vi "Modbus Master Example.vi"() -> ()   [LabVIEW 2021]
doc: "An example of the modbus master functionality."
uses:
  API/Master/Modbus Master.lvclass
  Master Function Definition/Read Device ID code.ctl
  Data Model/Device Data Model.lvclass
  API/Wrapper/API Main.lvlib
panel:
  in  "Stop Button":bool
  in  "Port":u16=502
  in  "Set Holding Registers":bool
  in  "Set Coils":bool
  in  "Fetch Discrete Inputs":bool
  in  "Fetch Input Registers":bool
  in  "Fetch Basic Objects":bool
  out "Basic Objects":string[](array[string])
  out "Status":string
  in  "Disconnect":bool
  in  "Connect":bool
  in  "Holding Registers":u16[](array[numeric])=[0, 0, 0, 0, 0, 0, 0, 0]
  out "Input Registers":u16[](array[numeric])
  in  "Coils":bool[](array[boolean])=[FALSE, FALSE, FALSE, FALSE, FALSE, FALSE, FALSE, FALSE]
  out "Discrete Inputs":bool[](array[boolean])
  in  "Slave Address":string="localhost"
  # "Coils are the boolean outputs of a modbus device. This example allows you to set the first 8 outputs."
  # "Holding Registers are the integer outputs of a modbus device. This example allows you to set the first 8 outputs."
  # "Modbus devices can also store objects in their memory, which are variable length strings. This example requests the basic level of objects."
  # "Discrete inputs are the boolean inputs of a modbus device. This example allows you to read the first 8 inputs."
  # "Input Registers are the integer inputs of a modbus device. This example allows you to read the first 8 inputs."
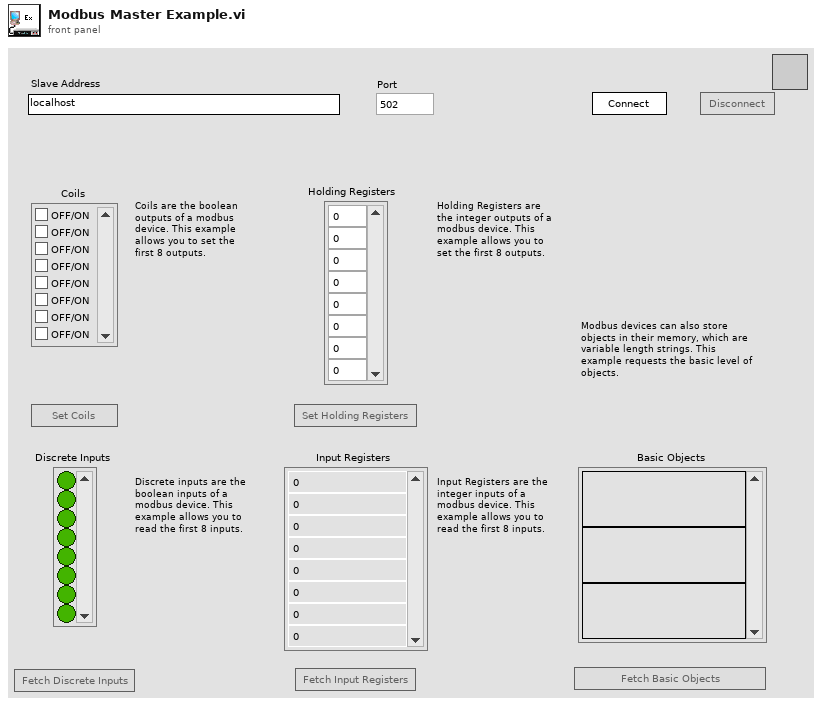
[diagram p1: front panel]
types:
  T1 = enum8{"Enabled", "Disabled", "Disabled and Grayed Out"}
  T2 = typedef "Device Data Model.lvclass/Read Device ID code.ctl" = enum8{"Read Basic", "Read Regular", "Read Extended", "Read Specific"}
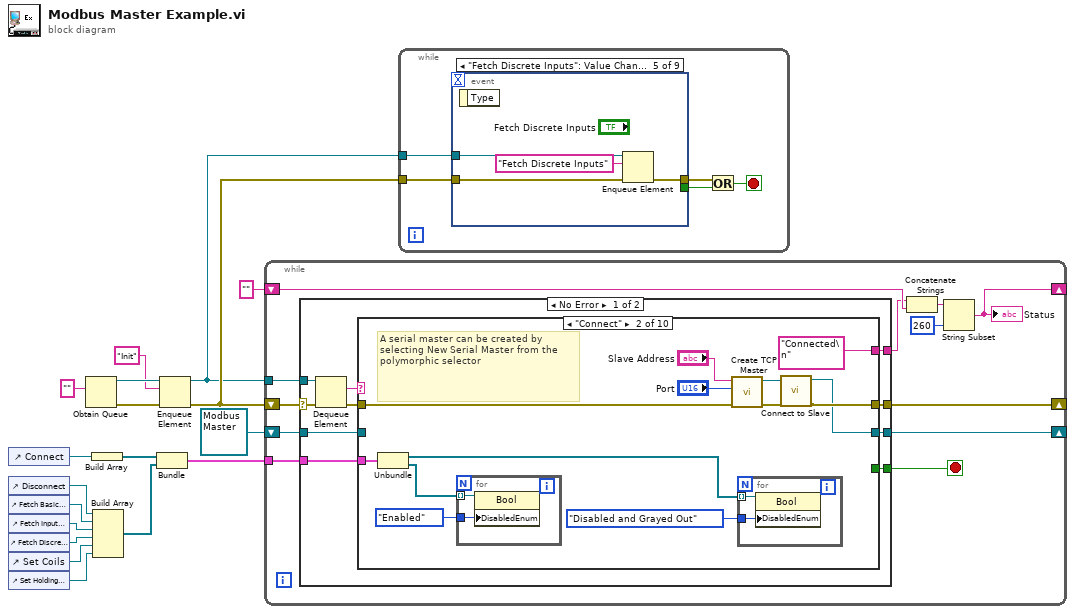
[diagram p0: block diagram]
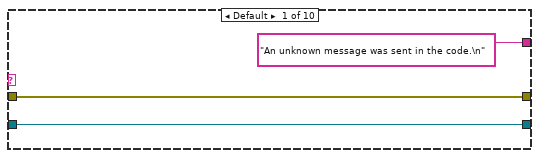
[diagram p2: hidden frame]
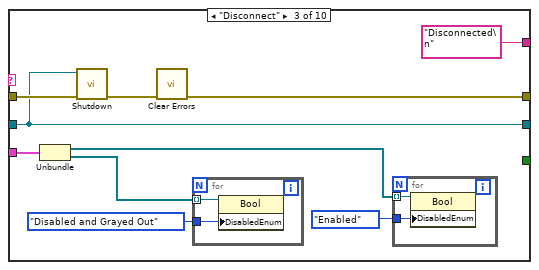
[diagram p3: hidden frame]
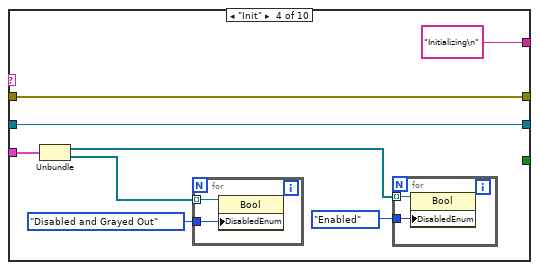
[diagram p4: hidden frame]
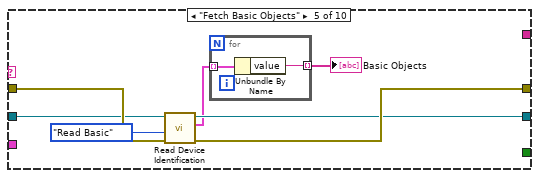
[diagram p5: hidden frame]
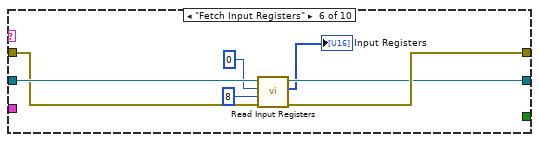
[diagram p6: hidden frame]
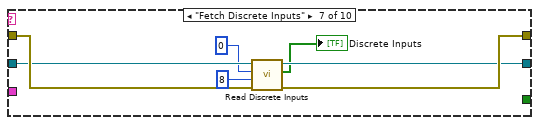
[diagram p7: hidden frame]
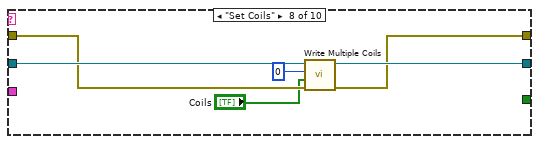
[diagram p8: hidden frame]
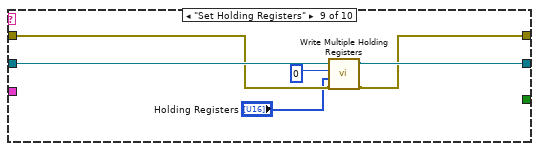
[diagram p9: hidden frame]
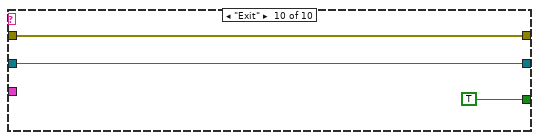
[diagram p10: hidden frame]
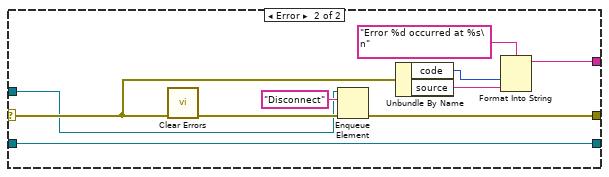
[diagram p11: hidden frame]
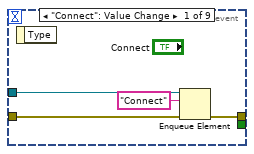
[diagram p12: hidden frame]
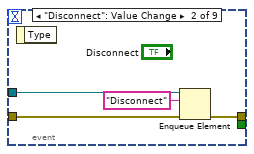
[diagram p13: hidden frame]
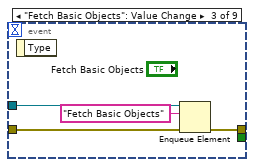
[diagram p14: hidden frame]
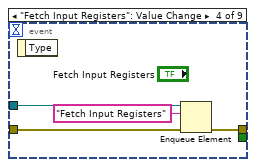
[diagram p15: hidden frame]
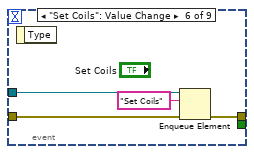
[diagram p16: hidden frame]
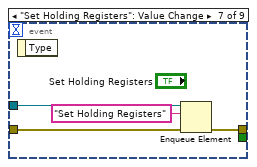
[diagram p17: hidden frame]
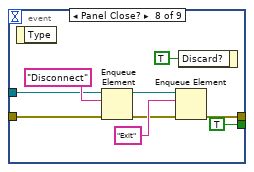
[diagram p18: hidden frame]
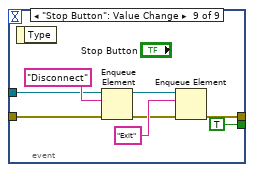
[diagram p19: hidden frame]
diagram:
  n1 = control-ref of="Connect"() -> (w9:refnum<vi>)
  n2 = control-ref of="Disconnect"() -> (w15:refnum<vi>)
  n3 = control-ref of="Fetch Basic Objects"() -> (w14:refnum<vi>)
  n4 = control-ref of="Fetch Input Registers"() -> (w13:refnum<vi>)
  n5 = control-ref of="Fetch Discrete Inputs"() -> (w12:refnum<vi>)
  n6 = control-ref of="Set Coils"() -> (w11:refnum<vi>)
  n7 = control-ref of="Set Holding Registers"() -> (w10:refnum<vi>)
  n8 = Obtain Queue(element data type="") -> (queue out=w4:refnum<queue>, error out=w18:errorcluster)  [unwired: 4 in, 1 out]
  n9 = Build Array(w9) -> (w6:refnum<vi>[])
  n10 = Build Array(w15, w14, w13, w12, w11, w10) -> (w8:refnum<vi>[])
  n11 = Bundle(w6, w8) -> (w7:cluster{refnum<vi>[], refnum<vi>[]})  [unwired: 1 in]
  n12 = Enqueue Element(queue=w4, element="Init", error in (no error)=w18) -> (queue out=w3:refnum<queue>, error out=w5:errorcluster)  [unwired: 1 in, 1 out]
  n13 = while {
    shift-right: [w22] -> _
    shift-left: refnum<class "Modbus Master.lvclass"> refnum ("Modbus Master") -> [w21]
    tunnel: w3 -> [w30]
    shift-right: [w28] -> _
    shift-left: w5 -> [w29]
    shift-right: [w27] -> _
    shift-left: "" ("Status") -> [w24]
    tunnel: w7 -> [w19]
    stop <- w20 stop-if-true
    n14 = case shown="No Error" w29 {
      selector: w29 -> [w39 w132]
      tunnel: w30 -> [w40 w126]
      tunnel: [w36 w133] -> w28
      tunnel: [w33 w129] -> w23
      tunnel: [w35 w125] -> w22
      tunnel: w21 -> [w34 w125]
      tunnel: [w32 _] -> w20
      tunnel: w19 -> [w31 _]
      frame No Error {
        n15 = Dequeue Element(queue=w40, error in (no error)=w39) -> (element=w37:string, error out=w38:errorcluster)  [unwired: 1 in, 2 out]
        n16 = case shown="\"Connect\"" w37 {
          tunnel: w38 -> [w43 w55 w70 w82 w93 w99 w109 w112 w118 w124]
          tunnel: [w43 w46 w66 w82 w92 w102 w108 w113 w119 w124] -> w36
          tunnel: [w42 w44 w68 w81 w90 w101 w106 w114 w120 w123] -> w35
          tunnel: w34 -> [w42 _ w68 w81 w91 w100 w107 w115 w121 w123]
          tunnel: ["An unknown message was sent in the code.\n" "Connected\n" "Disconnected\n" "Initializing\n" _ _ _ _ _ _] -> w33
          tunnel: [_ _ _ _ _ _ _ _ _ TRUE] -> w32
          tunnel: w31 -> [_ w53 w65 w79 _ _ _ _ _ _]
          frame Default {
          }
          frame "Connect" {
            # "A serial master can be created by selecting New Serial Master from the polymorphic selector"
            n17 = Unbundle(w53) -> (w51:refnum<vi>[], w52:refnum<vi>[])
            n18 = for {
              tunnel: w52 -> [w58] mode=indexing
              tunnel: T1."Enabled" ("Disabled") -> [w57]
              n19 = property class="Bool"(reference=w58, "DisabledEnum"=w57) -> ()  [unwired: 1 in, 2 out]
            }
            n20 = call "Create TCP Master.vi"("error in"=w55, "port (502)"="Port", "address"="Slave Address") -> ("error out"=w47:errorcluster, "TCP master instance"=w45:refnum<class "Modbus Master.lvclass">)  [unwired: 7 in]
            n21 = for {
              tunnel: w51 -> [w60] mode=indexing
              tunnel: T1."Disabled and Grayed Out" ("Disabled") -> [w59]
              n22 = property class="Bool"(reference=w60, "DisabledEnum"=w59) -> ()  [unwired: 1 in, 2 out]
            }
            n23 = call-dynamic "Connect to Slave.vi"("error in (no error)"=w47, "Modbus master in"=w45) -> ("error out"=w46:errorcluster, "Modbus master out"=w44:refnum<class "Modbus Master.lvclass">)  [unwired: 8 in]
          }
          frame "Disconnect" {
            n24 = Unbundle(w65) -> (w63:refnum<vi>[], w64:refnum<vi>[])
            n25 = call-dynamic "Shutdown.vi"("error in"=w70, "Modbus instance in"=w68) -> ("error out"=w69:errorcluster)  [unwired: 9 in]
            n26 = call <vilib>:"Clear Errors.vi"("error in (no error)"=w69) -> ("error out"=w66:errorcluster)  [unwired: 5 in, 1 out]
            n27 = for {
              tunnel: w64 -> [w74] mode=indexing
              tunnel: T1."Disabled and Grayed Out" ("Disabled") -> [w73]
              n28 = property class="Bool"(reference=w74, "DisabledEnum"=w73) -> ()  [unwired: 1 in, 2 out]
            }
            n29 = for {
              tunnel: w63 -> [w72] mode=indexing
              tunnel: T1."Enabled" ("Disabled") -> [w71]
              n30 = property class="Bool"(reference=w72, "DisabledEnum"=w71) -> ()  [unwired: 1 in, 2 out]
            }
          }
          frame "Init" {
            n31 = Unbundle(w79) -> (w77:refnum<vi>[], w78:refnum<vi>[])
            n32 = for {
              tunnel: w78 -> [w86] mode=indexing
              tunnel: T1."Disabled and Grayed Out" ("Disabled") -> [w85]
              n33 = property class="Bool"(reference=w86, "DisabledEnum"=w85) -> ()  [unwired: 1 in, 2 out]
            }
            n34 = for {
              tunnel: w77 -> [w84] mode=indexing
              tunnel: T1."Enabled" ("Disabled") -> [w83]
              n35 = property class="Bool"(reference=w84, "DisabledEnum"=w83) -> ()  [unwired: 1 in, 2 out]
            }
          }
          frame "Fetch Basic Objects" {
            n36 = call-dynamic "Read Device Identification.vi"("error in (no error)"=w93, "read device ID code"=Read_Device_ID_code."Read Basic" ("Read Device ID code"), "Modbus master in"=w91) -> ("error out"=w92:errorcluster, "objects"=w88:cluster{"object ID":u8, "value":string}[], "Modbus master out"=w90:refnum<class "Modbus Master.lvclass">)  [unwired: 6 in]
            n37 = for {
              tunnel: w88 -> [w95] mode=indexing
              tunnel: [w94] -> w87 mode=indexing
              n38 = Unbundle By Name(w95) -> ("value"=w94:string)
            }
            "Basic Objects" <- w87
          }
          frame "Fetch Input Registers" {
            n39 = call-dynamic "Read Input Registers.vi"("error in (no error)"=w99, "number of input registers"=u16 8 ("number of registers"), "starting address"=u16 0, "Modbus master in"=w100) -> ("error out"=w102:errorcluster, "register values"=→"Input Registers":u16[], "Modbus master out"=w101:refnum<class "Modbus Master.lvclass">)  [unwired: 5 in]
          }
          frame "Fetch Discrete Inputs" {
            n40 = call-dynamic "Read Discrete Inputs.vi"("error in (no error)"=w109, "number of discrete inputs"=u16 8 ("number of inputs"), "starting address"=u16 0, "Modbus master in"=w107) -> ("error out"=w108:errorcluster, "discrete input values"=→"Discrete Inputs":bool[], "Modbus master out"=w106:refnum<class "Modbus Master.lvclass">)  [unwired: 5 in]
          }
          frame "Set Coils" {
            n41 = call-dynamic "Write Multiple Coils.vi"("error in (no error)"=w112, "coil values"="Coils", "starting address"=u16 0, "Modbus master in"=w115) -> ("error out"=w113:errorcluster, "Modbus master out"=w114:refnum<class "Modbus Master.lvclass">)  [unwired: 6 in]
          }
          frame "Set Holding Registers" {
            n42 = call-dynamic "Write Multiple Holding Registers.vi"("error in (no error)"=w118, "holding register values"="Holding Registers", "starting address"=u16 0, "Modbus master in"=w121) -> ("error out"=w119:errorcluster, "Modbus master out"=w120:refnum<class "Modbus Master.lvclass">)  [unwired: 6 in]
          }
          frame "Exit" {
          }
        }
      }
      frame Error {
        n43 = call <vilib>:"Clear Errors.vi"("error in (no error)"=w132) -> ("error out"=w134:errorcluster)  [unwired: 5 in, 1 out]
        n44 = Enqueue Element(queue=w126, element="Disconnect", error in (no error)=w134) -> (error out=w133:errorcluster)  [unwired: 1 in, 2 out]
        n45 = Unbundle By Name(w132) -> ("code"=w131:i32, "source"=w130:string)
        n46 = Format Into String(format string="Error %d occurred at %s\n", w131, w130) -> (resulting string=w129:string)  [unwired: 2 in, 1 out]
      }
    }
    n47 = Concatenate Strings(w23, w24) -> (w25:string)
    n48 = String Subset(string=w25, length (rest)=260 ("length (rest)")) -> (substring=w27:string)  [unwired: 1 in]
    "Status" <- w27
  }
  n49 = while {
    tunnel: w5 -> [w139]
    tunnel: w3 -> [w138]
    stop <- w135 stop-if-true
    n50 = event shown="[4] \"Fetch Discrete Inputs\": Value Change" {
      selector: _ -> [_ _ _ _ _ _ _ _ _]
      dyn-events: _ -> [_ _ _ _ _ _ _ _ _]
      timeout: _ -> [_ _ _ _ _ _ _ _ _]
      tunnel: w139 -> [w143 w147 w151 w155 w159 w163 w167 w173 w182]
      tunnel: [w142 w146 w150 w154 w158 w162 w166 w168 w177] -> w137
      tunnel: w138 -> [w141 w145 w149 w153 w157 w161 w165 w170 w179]
      tunnel: [_ _ _ _ _ _ _ TRUE ("Discard?") TRUE ("Discard?")] -> w136
      event "Connect": Value Change {
        n51 = event-data() -> ()  [unwired: 1 in, 1 out]
        n52 = Enqueue Element(queue=w141, element="Connect", error in (no error)=w143) -> (error out=w142:errorcluster)  [unwired: 1 in, 2 out]
      }
      event "Disconnect": Value Change {
        n53 = event-data() -> ()  [unwired: 1 in, 1 out]
        n54 = Enqueue Element(queue=w145, element="Disconnect", error in (no error)=w147) -> (error out=w146:errorcluster)  [unwired: 1 in, 2 out]
      }
      event "Fetch Basic Objects": Value Change {
        n55 = event-data() -> ()  [unwired: 1 in, 1 out]
        n56 = Enqueue Element(queue=w149, element="Fetch Basic Objects", error in (no error)=w151) -> (error out=w150:errorcluster)  [unwired: 1 in, 2 out]
      }
      event "Fetch Input Registers": Value Change {
        n57 = event-data() -> ()  [unwired: 1 in, 1 out]
        n58 = Enqueue Element(queue=w153, element="Fetch Input Registers", error in (no error)=w155) -> (error out=w154:errorcluster)  [unwired: 1 in, 2 out]
      }
      event "Fetch Discrete Inputs": Value Change {
        n59 = event-data() -> ()  [unwired: 1 in, 1 out]
        n60 = Enqueue Element(queue=w157, element="Fetch Discrete Inputs", error in (no error)=w159) -> (error out=w158:errorcluster)  [unwired: 1 in, 2 out]
      }
      event "Set Coils": Value Change {
        n61 = event-data() -> ()  [unwired: 1 in, 1 out]
        n62 = Enqueue Element(queue=w161, element="Set Coils", error in (no error)=w163) -> (error out=w162:errorcluster)  [unwired: 1 in, 2 out]
      }
      event "Set Holding Registers": Value Change {
        n63 = event-data() -> ()  [unwired: 1 in, 1 out]
        n64 = Enqueue Element(queue=w165, element="Set Holding Registers", error in (no error)=w167) -> (error out=w166:errorcluster)  [unwired: 1 in, 2 out]
      }
      event Panel Close? {
        n65 = event-data() -> ()  [unwired: 1 in, 1 out]
        n66 = Enqueue Element(queue=w170, element="Disconnect", error in (no error)=w173) -> (queue out=w171:refnum<queue>, error out=w169:errorcluster)  [unwired: 1 in, 1 out]
        n67 = Enqueue Element(queue=w171, element="Exit", error in (no error)=w169) -> (error out=w168:errorcluster)  [unwired: 1 in, 2 out]
        n68 = event-data("Discard?"=TRUE) -> ()  [unwired: 1 in, 1 out]
      }
      event "Stop Button": Value Change {
        n69 = event-data() -> ()  [unwired: 1 in, 1 out]
        n70 = Enqueue Element(queue=w179, element="Disconnect", error in (no error)=w182) -> (queue out=w180:refnum<queue>, error out=w178:errorcluster)  [unwired: 1 in, 1 out]
        n71 = Enqueue Element(queue=w180, element="Exit", error in (no error)=w178) -> (error out=w177:errorcluster)  [unwired: 1 in, 2 out]
      }
    }
    n72 = Or(x=w137, y=w136) -> (x .or. y?=w135:bool)
  }
